vi "Initiate Pattern Generation.vi"(0 "NI Digital in":refnum<k15>, 5 "Trigger Configuration":T1={"Burst Trigger Type"=1700, "Digital Edge Source"="PXI_Trig0", "Digital Edge Type"=1800} {"Digital Edge Type" items=["Rising Edge"=1800, "Falling Edge"=1801]; "Burst Trigger Type" items=["None"=1700, "Digital Edge"=1701, "Software"=1702]}, 7 "Pattern Start Label":string, 11 "error in (no error)":errorcluster) -> (4 "NI Digital out":refnum<k15>, 15 "error out":errorcluster)   [LabVIEW 2016, in "Digital.lvlib"]
uses:
  Digital.lvlib
  <instrlib>/niDigital/niDigital.llb/niDigital Burst Pattern (Burst Only).vi
  <instrlib>/niDigital/niDigital.llb/niDigital Configure Software Edge Start Trigger.vi
  <instrlib>/niDigital/niDigital.llb/niDigital Configure Digital Edge Start Trigger.vi
  <instrlib>/niDigital/niDigital.llb/niDigital Disable Start Trigger.vi
  <instrlib>/niDigital/niDigital.llb/niDigital Trigger Terminals.ctl
  <instrlib>/niDigital/niDigital.llb/niDigital Trigger Digital Edge - Edge.ctl
  Type Definitions/Trigger Configuration.ctl
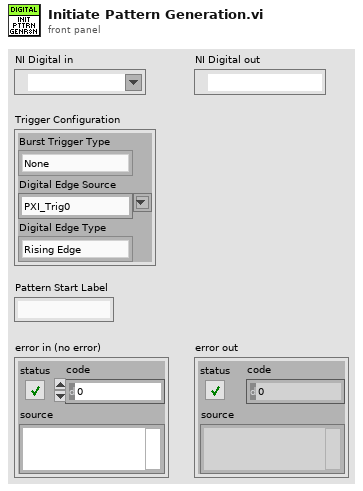
[diagram p1: front panel]
types:
  T1 = typedef "Digital.lvlib/Trigger Configuration.ctl" = cluster{"Burst Trigger Type":i32, "Digital Edge Source":T2, "Digital Edge Type":T3}
  T2 = typedef "niDigital Trigger Terminals.ctl" = string
  T3 = typedef "niDigital Trigger Digital Edge - Edge.ctl" = i32
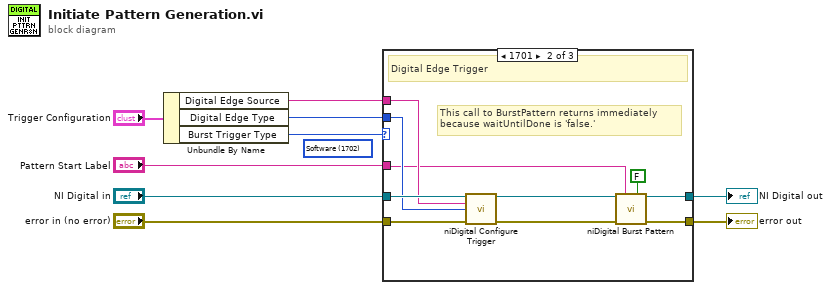
[diagram p0: block diagram]
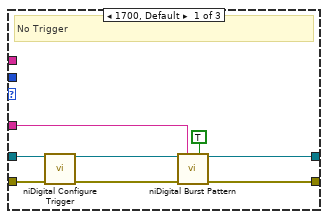
[diagram p2: hidden frame]
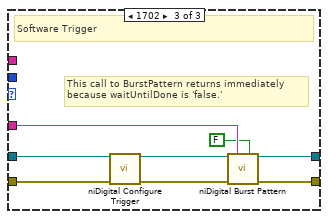
[diagram p3: hidden frame]
diagram:
  (unwired) 1702 items=["None"=1700, "Digital Edge"=1701, "Software"=1702] ("Burst Trigger Type")
  n1 = Unbundle By Name("Trigger Configuration") -> ("Digital Edge Source"=w2:T2, "Digital Edge Type"=w1:T3, "Burst Trigger Type"=w4:i32)
  n2 = case shown="1701" w4 {
    tunnel: "error in (no error)" -> [w17 w27 w35]
    tunnel: [w14 w22 w32] -> w7
    tunnel: "NI Digital in" -> [w15 w25 w33]
    tunnel: [w12 w20 w30] -> w5
    tunnel: "Pattern Start Label" -> [w11 w19 w29]
    tunnel: w2 -> [_ w24 _]
    tunnel: w1 -> [_ w23 _]
    frame 1700, Default {
      # "No Trigger"
      n3 = call-poly <instrlib>:"niDigital Configure Trigger.vi"("instrument handle"=w15, "error in"=w17) -> ("instrument handle out"=w13:refnum<k15>, "error out"=w16:errorcluster)  [unwired: 12 in]
      n4 = call-poly <instrlib>:"niDigital Burst Pattern.vi"("instrument handle"=w13, "start label"=w11, "wait until done? (T)"=TRUE, "error in"=w16) -> ("instrument handle out"=w12:refnum<k15>, "error out"=w14:errorcluster)  [unwired: 10 in]
    }
    frame 1701 {
      # "This call to BurstPattern returns immediately because waitUntilDone is 'false.'"
      # "Digital Edge Trigger"
      n5 = call-poly <instrlib>:"niDigital Configure Trigger.vi"("instrument handle"=w25, "source"=w24, "edge"=w23, "error in"=w27) -> ("instrument handle out"=w21:refnum<k15>, "error out"=w26:errorcluster)  [unwired: 10 in]
      n6 = call-poly <instrlib>:"niDigital Burst Pattern.vi"("instrument handle"=w21, "start label"=w19, "wait until done? (T)"=FALSE, "error in"=w26) -> ("instrument handle out"=w20:refnum<k15>, "error out"=w22:errorcluster)  [unwired: 10 in]
    }
    frame 1702 {
      # "This call to BurstPattern returns immediately because waitUntilDone is 'false.'"
      # "Software Trigger"
      n7 = call-poly <instrlib>:"niDigital Configure Trigger.vi"("instrument handle"=w33, "error in"=w35) -> ("instrument handle out"=w31:refnum<k15>, "error out"=w34:errorcluster)  [unwired: 12 in]
      n8 = call-poly <instrlib>:"niDigital Burst Pattern.vi"("instrument handle"=w31, "start label"=w29, "wait until done? (T)"=FALSE, "error in"=w34) -> ("instrument handle out"=w30:refnum<k15>, "error out"=w32:errorcluster)  [unwired: 10 in]
    }
  }
  "NI Digital out" <- w5
  "error out" <- w7
